vi "Volatus Type Lookup.vi"(7 "Don't Recurse Past Match (F)":bool, 8 "error in (no error)":errorcluster, 10 "Meta Type":T1=enum."VL_System", 11 "Config Lookup (New)":refnum<class "Config Lookup.lvclass">) -> (0 "error out":errorcluster, 3 "Config Lookup out":refnum<class "Config Lookup.lvclass">)   [LabVIEW 2020, in "VolatusConfig.lvlib"]
uses:
  VolatusConfig.lvlib
  lv-cdm/CDM-Config/Config Filter/Config Lookup.lvclass
  Meta Type.ctl
  Meta Name.ctl
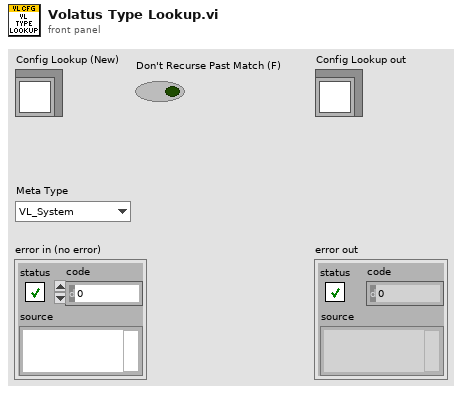
[diagram p1: front panel]
types:
  T1 = typedef "VolatusConfig.lvlib/Meta Type.ctl" = enum16{"UNKNOWN", "VL_System", "VL_Cluster", "VL_Node", "VL_Task", "VL_Group", "VL_Channel", "VL_Task_List", "VL_Scaling", "VL_Sensor", "VL_Sensor_List", "VL_Scale"}
  T2 = typedef "VolatusConfig.lvlib/Meta Name.ctl" = enum16{"VL_Type", "VL_Node_IP", "VL_Node_Type", "VL_Task_Type", "VL_Group_Type", "VL_Channel_Type", "VL_Channel_DataType", "VL_Config_Version", "VL_Overlay_Type"}
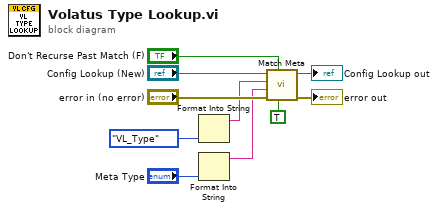
[diagram p0: block diagram]
diagram:
  n1 = Format Into String(Meta_Name."VL_Type" ("Meta Name")) -> (resulting string=w5:string)  [unwired: 3 in, 1 out]
  n2 = Format Into String("Meta Type") -> (resulting string=w3:string)  [unwired: 3 in, 1 out]
  n3 = call "Match Meta.vi"("Exact Value (F)"=TRUE, "Don't Recurse Past Match (F)"="Don't Recurse Past Match (F)", "error in (no error)"="error in (no error)", "Value (Any)"=w3, "Name"=w5, "Config Lookup (New)"="Config Lookup (New)") -> ("error out"=→"error out":errorcluster, "Config Lookup out"=→"Config Lookup out":refnum<class "Config Lookup.lvclass">)  [unwired: 4 in]
